vi "QCA - DUT Get Rx PSR.vi"(8 "error in (no error)":errorcluster, 11 "CART TCP Connection In":refnum<k5>) -> (0 "error out":errorcluster, 2 "Correct Frames":i32, 3 "CART TCP Connection Out":refnum<k5>)   [LabVIEW 2012]
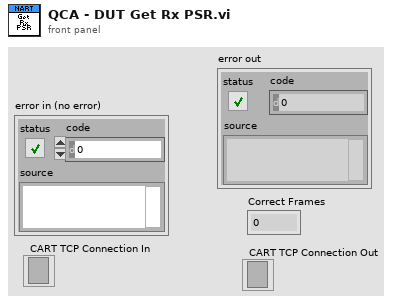
[diagram p1: front panel]
types:
  T1 = cluster{"Correct Frames":i32, "Throughput":i32, "Error":i32}
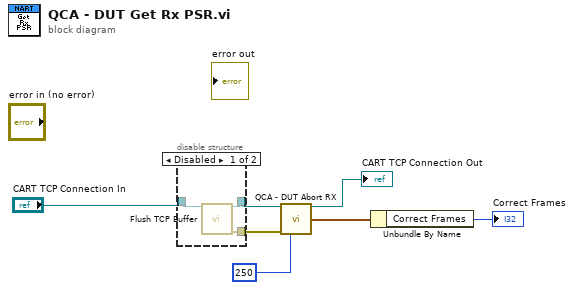
[diagram p0: block diagram]
diagram:
  n1 = disable-structure shown="Disabled" {
    disable-tunnel: [w10 w11] -> w6
    disable-tunnel: [w9 _] -> w5
    disable-tunnel: "CART TCP Connection In" -> [w8 w11]
    frame Disabled {
      n2 = call "Flush TCP Buffer.vi"("CART TCP Connection In"=w8) -> ("CART TCP Connection Out"=w10:refnum<k5>, "error out"=w9:errorcluster)  [unwired: 13 in]
    }
    frame Enabled {
    }
  }
  n3 = call "QCA - DUT Abort RX.vi"("CART TCP Connection In"=w6, "error in (no error)"=w5, "Read Time Out(ms)"=250) -> ("CART TCP Connection Out"=→"CART TCP Connection Out":refnum<k5>, "TX Response"=w4:T1)  [unwired: 10 in, 1 out]
  n4 = Unbundle By Name(w4) -> ("Correct Frames"=→"Correct Frames":i32)
